vi "1.Primary Interface.vi"() -> ()   [LabVIEW 2020]
uses:
  UnderAutomation.UniversalRobots/UnderAutomation.UniversalRobots.lvlib
  C:/Users/fg/Documents/UniversalRobots.vi/LabVIEW_2024/UnderAutomation.UniversalRobots/lib/UnderAutomation.UniversalRobots.dll
  LabVIEW_2024/UnderAutomation.UniversalRobots/lib/UnderAutomation.UniversalRobots.dll
panel:
  out "UR Robot":refnum<k24>
  out "PrimaryInterface":refnum<k24>
  out "Connected":bool
  in  "Tab Control":T1(tab)
  in  "Disconnect":bool
  in  "Test":bool
  in  "Key":string
  in  "Licensee":string
  in  "Connect":bool
  in  "IP":string caption="Robot IP Address"
  out "License state":string
  out "Connect error":string
  in  "Script":string
  in  "Send":bool
  out "Variables":T2(array[cluster])
  out "CartesianInfo":T3
  out "ForceModeData":T4
  out "JointData":T5
  out "ToolData":T6
  out "AdditionalInfo":T7
  out "ToolCommunicationInfo":T8
  out "MasterboardData":T9
  out "ToolModeInfo":T10
  out "RobotModeData":T11
  out "TextMessage":cluster{"TextMessage":string}
  out "KeyMessage":T12
  out "PopupMessage":T13
  out "RuntimeExceptionMessage":T14
  out "KinematicsInfo":T15
  out "CalibrationData":T16
  out "SingularityInfo":T17
  out "ConfigurationData":T18
  out "Version":T19
  in  "stop":bool
  # "UnderAutomation"
  # "https://underautomation.com/universal-robots"
  # "+"
  # "LabVIEW demo app for remote control and monitoring of your Universal Robots cobot"
  # "Connect to robot"
  # "2. Ensure you have a trial or lifetime valid license"
  # "1. Set UR cobot address"
  # "This is a commercial library, you have a 30-day trial period. But you can use it forever if you buy a perpetual licence for your company (regardless of the number of robot, applications or developers)."
  # "If you have a license :"
  # "2. Connect to the robot"
  # "Send script"
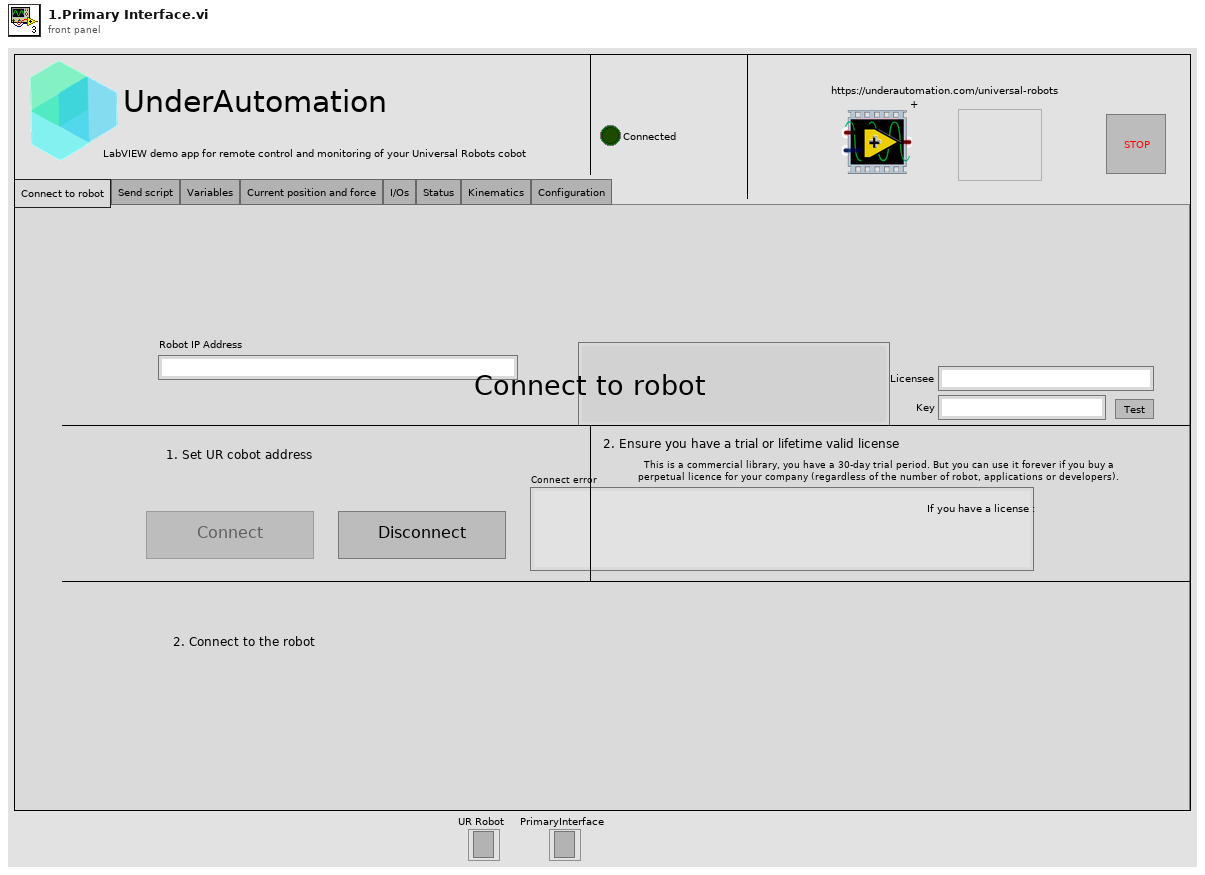
[diagram p1: front panel]
types:
  T1 = enum32{"Connect to robot", "Send script", "Variables", "Current position and force", "I/Os", "Status", "Kinematics", "Configuration"}
  T2 = cluster{"Name":string, "Milliseconds":i32, "Type":i32, "BoolValue":bool, "FloatValue":sgl, "IntValue":i32, "StringValue":string, "PoseValue":cluster{"X":dbl, "Y":dbl, "Z":dbl, "Rx":dbl, "Ry":dbl, "Rz":dbl}}[]
  T3 = cluster{"X":dbl, "Y":dbl, "Z":dbl, "Rx":dbl, "Ry":dbl, "Rz":dbl, "TCPOffsetX":dbl, "TCPOffsetY":dbl, "TCPOffsetZ":dbl, "TCPOffsetRX":dbl, "TCPOffsetRY":dbl, "TCPOffsetRZ":dbl}
  T4 = cluster{"X":dbl, "Y":dbl, "Z":dbl, "Rx":dbl, "Ry":dbl, "Rz":dbl, "RobotDexterity":dbl}
  T5 = cluster{"Base":cluster{"ActualSpeed":dbl, "Current":sgl, "JointMode":u8, "Position":dbl, "TargetPosition":dbl, "Temperature":sgl, "Voltage":sgl}, "Shoulder":cluster{"ActualSpeed":dbl, "Current":sgl, "JointMode":u8, "Position":dbl, "TargetPosition":dbl, "Temperature":sgl, "Voltage":sgl}, "Elbow":cluster{"ActualSpeed":dbl, "Current":sgl, "JointMode":u8, "Position":dbl, "TargetPosition":dbl, "Temperature":sgl, "Voltage":sgl}, "Wrist1":cluster{"ActualSpeed":dbl, "Current":sgl, "JointMode":u8, "Position":dbl, "TargetPosition":dbl, "Temperature":sgl, "Voltage":sgl}, "Wrist2":cluster{"ActualSpeed":dbl, "Current":sgl, "JointMode":u8, "Position":dbl, "TargetPosition":dbl, "Temperature":sgl, "Voltage":sgl}, "Wrist3":cluster{"ActualSpeed":dbl, "Current":sgl, "JointMode":u8, "Position":dbl, "TargetPosition":dbl, "Temperature":sgl, "Voltage":sgl}}
  T6 = cluster{"AnalogInput2":dbl, "AnalogInput3":dbl, "AnalogInputRange2":i32, "AnalogInputRange3":i32, "ToolCurrent":sgl, "ToolMode":u8, "ToolOutputVoltage":i8, "ToolTemperature":sgl, "ToolVoltage48V":sgl}
  T7 = cluster{"FreedriveButtonEnabled":bool, "FreedriveButtonPressed":bool, "IOEnabledFreedrive":bool}
  T8 = cluster{"BaudRate":i32, "Parity":i32, "RxIdleChars":sgl, "TxIdleChars":sgl, "ToolCommunicationIsEnabled":bool, "StopBits":i32}
  T9 = cluster{"AnalogInput0":dbl, "AnalogInput1":dbl, "AnalogInputRange0":i32, "AnalogInputRange1":i32, "AnalogOutput0":dbl, "AnalogOutput1":dbl, "AnalogOutputDomain0":i32, "AnalogOutputDomain1":i32, "DigitalInputs":cluster{"Configurable0":bool, "Configurable1":bool, "Configurable2":bool, "Configurable3":bool, "Configurable4":bool, "Configurable5":bool, "Configurable6":bool, "Configurable7":bool, "Digital0":bool, "Digital1":bool, "Digital2":bool, "Digital3":bool, "Digital4":bool, "Digital5":bool, "Digital6":bool, "Digital7":bool, "ToolDigital0":bool, "ToolDigital1":bool, "Value":i32}, "DigitalOutputs":cluster{"Configurable0":bool, "Configurable1":bool, "Configurable2":bool, "Configurable3":bool, "Configurable4":bool, "Configurable5":bool, "Configurable6":bool, "Configurable7":bool, "Digital0":bool, "Digital1":bool, "Digital2":bool, "Digital3":bool, "Digital4":bool, "Digital5":bool, "Digital6":bool, "Digital7":bool, "ToolDigital0":bool, "ToolDigital1":bool, "Value":i32}, "Euromap67Installed":i8, "EuromapCurrent":sgl, "EuromapInputBits":i32, "EuromapOutputBits":i32, "EuromapVoltage":sgl, "InReducedMode":u8, "MasterboardTemperature":sgl, "MasterIOCurrent":sgl, "OperationalModeSelectorInput":u8, "RobotCurrent":sgl, "RobotVoltage48V":sgl, "Safetymode":u8, "ThreePositionEnablingDeviceInput":u8}
  T10 = cluster{"DigitalOutputMode0":i32, "DigitalOutputMode1":i32, "OutputMode":i32}
  T11 = cluster{"ControlMode":i32, "EmergencyStopped":bool, "PhysicalRobotConnected":bool, "ProgramPaused":bool, "ProgramRunning":bool, "ProtectiveStopped":bool, "RealRobotEnabled":bool, "RobotMode":i32, "RobotPowerOn":bool, "SpeedScaling":dbl, "TargetSpeedFraction":dbl, "TargetSpeedFractionLimit":dbl, "TotalMilliseconds":dbl}
  T12 = cluster{"KeyTextMessage":string, "RobotMessageArgument":i32, "RobotMessageCode":i32, "RobotMessageTitle":string}
  T13 = cluster{"Blocking":bool, "Error":bool, "PopupMessageTitle":string, "PopupTextMessage":string, "RequestedType":i32, "RequestId":u32, "Warning":bool}
  T14 = cluster{"RuntimeExceptionTextMessage":string, "ScriptColumnNumber":i32, "ScriptLineNumber":i32}
  T15 = cluster{"Base":cluster{"Checksum":i32, "DHa":dbl, "Dhalpha":dbl, "DHd":dbl, "DHtheta":dbl}, "Shoulder":cluster{"Checksum":i32, "DHa":dbl, "Dhalpha":dbl, "DHd":dbl, "DHtheta":dbl}, "Elbow":cluster{"Checksum":i32, "DHa":dbl, "Dhalpha":dbl, "DHd":dbl, "DHtheta":dbl}, "Wrist1":cluster{"Checksum":i32, "DHa":dbl, "Dhalpha":dbl, "DHd":dbl, "DHtheta":dbl}, "Wrist2":cluster{"Checksum":i32, "DHa":dbl, "Dhalpha":dbl, "DHd":dbl, "DHtheta":dbl}, "Wrist3":cluster{"Checksum":i32, "DHa":dbl, "Dhalpha":dbl, "DHd":dbl, "DHtheta":dbl}, "CalibrationStatus":i32}
  T16 = cluster{"Fx":dbl, "Fy":dbl, "Fz":dbl, "Frx":dbl, "Fry":dbl, "Frz":dbl}
  T17 = cluster{"SingularitySeverity":u8, "SingularityType":u8}
  T18 = cluster{"AJointDefault":dbl, "AToolDefault":dbl, "ControllerBoxType":i32, "EqRadius":dbl, "MasterboardVersion":i32, "RobotSubType":i32, "RobotType":i32, "VJointDefault":dbl, "VToolDefault":dbl, "Base":cluster{"DHa":dbl, "DHalpha":dbl, "DHd":dbl, "DHtheta":dbl, "JointMaxAcceleration":dbl, "JointMaxLimit":dbl, "JointMaxSpeed":dbl, "JointMinLimit":dbl}, "Shoulder":cluster{"DHa":dbl, "DHalpha":dbl, "DHd":dbl, "DHtheta":dbl, "JointMaxAcceleration":dbl, "JointMaxLimit":dbl, "JointMaxSpeed":dbl, "JointMinLimit":dbl}, "Elbow":cluster{"DHa":dbl, "DHalpha":dbl, "DHd":dbl, "DHtheta":dbl, "JointMaxAcceleration":dbl, "JointMaxLimit":dbl, "JointMaxSpeed":dbl, "JointMinLimit":dbl}, "Wrist1":cluster{"DHa":dbl, "DHalpha":dbl, "DHd":dbl, "DHtheta":dbl, "JointMaxAcceleration":dbl, "JointMaxLimit":dbl, "JointMaxSpeed":dbl, "JointMinLimit":dbl}, "Wrist2":cluster{"DHa":dbl, "DHalpha":dbl, "DHd":dbl, "DHtheta":dbl, "JointMaxAcceleration":dbl, "JointMaxLimit":dbl, "JointMaxSpeed":dbl, "JointMinLimit":dbl}, "Wrist3":cluster{"DHa":dbl, "DHalpha":dbl, "DHd":dbl, "DHtheta":dbl, "JointMaxAcceleration":dbl, "JointMaxLimit":dbl, "JointMaxSpeed":dbl, "JointMinLimit":dbl}}
  T19 = cluster{"MajorVersion":u8, "MinorVersion":u8, "BugfixVersion":i32, "BuildNumber":i32, "BuildDate":string, "ProjectName":string}
  T20 = enum8{"Enabled", "Disabled", "Disabled and Grayed Out"}
  T21 = cluster{"AdditionalInfo":cluster{"FreedriveButtonEnabled":bool, "FreedriveButtonPressed":bool, "IOEnabledFreedrive":bool}, "CalibrationData":cluster{"Fx":dbl, "Fy":dbl, "Fz":dbl, "Frx":dbl, "Fry":dbl, "Frz":dbl}, "CartesianInfo":cluster{"X":dbl, "Y":dbl, "Z":dbl, "Rx":dbl, "Ry":dbl, "Rz":dbl, "TCPOffsetX":dbl, "TCPOffsetY":dbl, "TCPOffsetZ":dbl, "TCPOffsetRX":dbl, "TCPOffsetRY":dbl, "TCPOffsetRZ":dbl}, "ConfigurationData":cluster{"AJointDefault":dbl, "AToolDefault":dbl, "ControllerBoxType":i32, "EqRadius":dbl, "MasterboardVersion":i32, "RobotSubType":i32, "RobotType":i32, "VJointDefault":dbl, "VToolDefault":dbl, "Base":cluster{"DHa":dbl, "DHalpha":dbl, "DHd":dbl, "DHtheta":dbl, "JointMaxAcceleration":dbl, "JointMaxLimit":dbl, "JointMaxSpeed":dbl, "JointMinLimit":dbl}, "Shoulder":cluster{"DHa":dbl, "DHalpha":dbl, "DHd":dbl, "DHtheta":dbl, "JointMaxAcceleration":dbl, "JointMaxLimit":dbl, "JointMaxSpeed":dbl, "JointMinLimit":dbl}, "Elbow":cluster{"DHa":dbl, "DHalpha":dbl, "DHd":dbl, "DHtheta":dbl, "JointMaxAcceleration":dbl, "JointMaxLimit":dbl, "JointMaxSpeed":dbl, "JointMinLimit":dbl}, "Wrist1":cluster{"DHa":dbl, "DHalpha":dbl, "DHd":dbl, "DHtheta":dbl, "JointMaxAcceleration":dbl, "JointMaxLimit":dbl, "JointMaxSpeed":dbl, "JointMinLimit":dbl}, "Wrist2":cluster{"DHa":dbl, "DHalpha":dbl, "DHd":dbl, "DHtheta":dbl, "JointMaxAcceleration":dbl, "JointMaxLimit":dbl, "JointMaxSpeed":dbl, "JointMinLimit":dbl}, "Wrist3":cluster{"DHa":dbl, "DHalpha":dbl, "DHd":dbl, "DHtheta":dbl, "JointMaxAcceleration":dbl, "JointMaxLimit":dbl, "JointMaxSpeed":dbl, "JointMinLimit":dbl}}, "ForceModeData":cluster{"X":dbl, "Y":dbl, "Z":dbl, "Rx":dbl, "Ry":dbl, "Rz":dbl, "RobotDexterity":dbl}, "JointData":cluster{"Base":cluster{"ActualSpeed":dbl, "Current":sgl, "JointMode":u8, "Position":dbl, "TargetPosition":dbl, "Temperature":sgl, "Voltage":sgl}, "Shoulder":cluster{"ActualSpeed":dbl, "Current":sgl, "JointMode":u8, "Position":dbl, "TargetPosition":dbl, "Temperature":sgl, "Voltage":sgl}, "Elbow":cluster{"ActualSpeed":dbl, "Current":sgl, "JointMode":u8, "Position":dbl, "TargetPosition":dbl, "Temperature":sgl, "Voltage":sgl}, "Wrist1":cluster{"ActualSpeed":dbl, "Current":sgl, "JointMode":u8, "Position":dbl, "TargetPosition":dbl, "Temperature":sgl, "Voltage":sgl}, "Wrist2":cluster{"ActualSpeed":dbl, "Current":sgl, "JointMode":u8, "Position":dbl, "TargetPosition":dbl, "Temperature":sgl, "Voltage":sgl}, "Wrist3":cluster{"ActualSpeed":dbl, "Current":sgl, "JointMode":u8, "Position":dbl, "TargetPosition":dbl, "Temperature":sgl, "Voltage":sgl}}, "KeyMessage":cluster{"KeyTextMessage":string, "RobotMessageArgument":i32, "RobotMessageCode":i32, "RobotMessageTitle":string}, "KinematicsInfo":cluster{"Base":cluster{"Checksum":i32, "DHa":dbl, "Dhalpha":dbl, "DHd":dbl, "DHtheta":dbl}, "Shoulder":cluster{"Checksum":i32, "DHa":dbl, "Dhalpha":dbl, "DHd":dbl, "DHtheta":dbl}, "Elbow":cluster{"Checksum":i32, "DHa":dbl, "Dhalpha":dbl, "DHd":dbl, "DHtheta":dbl}, "Wrist1":cluster{"Checksum":i32, "DHa":dbl, "Dhalpha":dbl, "DHd":dbl, "DHtheta":dbl}, "Wrist2":cluster{"Checksum":i32, "DHa":dbl, "Dhalpha":dbl, "DHd":dbl, "DHtheta":dbl}, "Wrist3":cluster{"Checksum":i32, "DHa":dbl, "Dhalpha":dbl, "DHd":dbl, "DHtheta":dbl}, "CalibrationStatus":i32}, "MasterboardData":cluster{"AnalogInput0":dbl, "AnalogInput1":dbl, "AnalogInputRange0":i32, "AnalogInputRange1":i32, "AnalogOutput0":dbl, "AnalogOutput1":dbl, "AnalogOutputDomain0":i32, "AnalogOutputDomain1":i32, "DigitalInputs":cluster{"Configurable0":bool, "Configurable1":bool, "Configurable2":bool, "Configurable3":bool, "Configurable4":bool, "Configurable5":bool, "Configurable6":bool, "Configurable7":bool, "Digital0":bool, "Digital1":bool, "Digital2":bool, "Digital3":bool, "Digital4":bool, "Digital5":bool, "Digital6":bool, "Digital7":bool, "ToolDigital0":bool, "ToolDigital1":bool, "Value":i32}, "DigitalOutputs":cluster{"Configurable0":bool, "Configurable1":bool, "Configurable2":bool, "Configurable3":bool, "Configurable4":bool, "Configurable5":bool, "Configurable6":bool, "Configurable7":bool, "Digital0":bool, "Digital1":bool, "Digital2":bool, "Digital3":bool, "Digital4":bool, "Digital5":bool, "Digital6":bool, "Digital7":bool, "ToolDigital0":bool, "ToolDigital1":bool, "Value":i32}, "Euromap67Installed":i8, "EuromapCurrent":sgl, "EuromapInputBits":i32, "EuromapOutputBits":i32, "EuromapVoltage":sgl, "InReducedMode":u8, "MasterboardTemperature":sgl, "MasterIOCurrent":sgl, "OperationalModeSelectorInput":u8, "RobotCurrent":sgl, "RobotVoltage48V":sgl, "Safetymode":u8, "ThreePositionEnablingDeviceInput":u8}, "PopupMessage":cluster{"Blocking":bool, "Error":bool, "PopupMessageTitle":string, "PopupTextMessage":string, "RequestedType":i32, "RequestId":u32, "Warning":bool}, "RobotModeData":cluster{"ControlMode":i32, "EmergencyStopped":bool, "PhysicalRobotConnected":bool, "ProgramPaused":bool, "ProgramRunning":bool, "ProtectiveStopped":bool, "RealRobotEnabled":bool, "RobotMode":i32, "RobotPowerOn":bool, "SpeedScaling":dbl, "TargetSpeedFraction":dbl, "TargetSpeedFractionLimit":dbl, "TotalMilliseconds":dbl}, "RuntimeExceptionMessage":cluster{"RuntimeExceptionTextMessage":string, "ScriptColumnNumber":i32, "ScriptLineNumber":i32}, "SingularityInfo":cluster{"SingularitySeverity":u8, "SingularityType":u8}, "TextMessage":cluster{"TextMessage":string}, "ToolCommunicationInfo":cluster{"BaudRate":i32, "Parity":i32, "RxIdleChars":sgl, "TxIdleChars":sgl, "ToolCommunicationIsEnabled":bool, "StopBits":i32}, "ToolData":cluster{"AnalogInput2":dbl, "AnalogInput3":dbl, "AnalogInputRange2":i32, "AnalogInputRange3":i32, "ToolCurrent":sgl, "ToolMode":u8, "ToolOutputVoltage":i8, "ToolTemperature":sgl, "ToolVoltage48V":sgl}, "ToolModeInfo":cluster{"DigitalOutputMode0":i32, "DigitalOutputMode1":i32, "OutputMode":i32}, "Version":cluster{"MajorVersion":u8, "MinorVersion":u8, "BugfixVersion":i32, "BuildNumber":i32, "BuildDate":string, "ProjectName":string}}
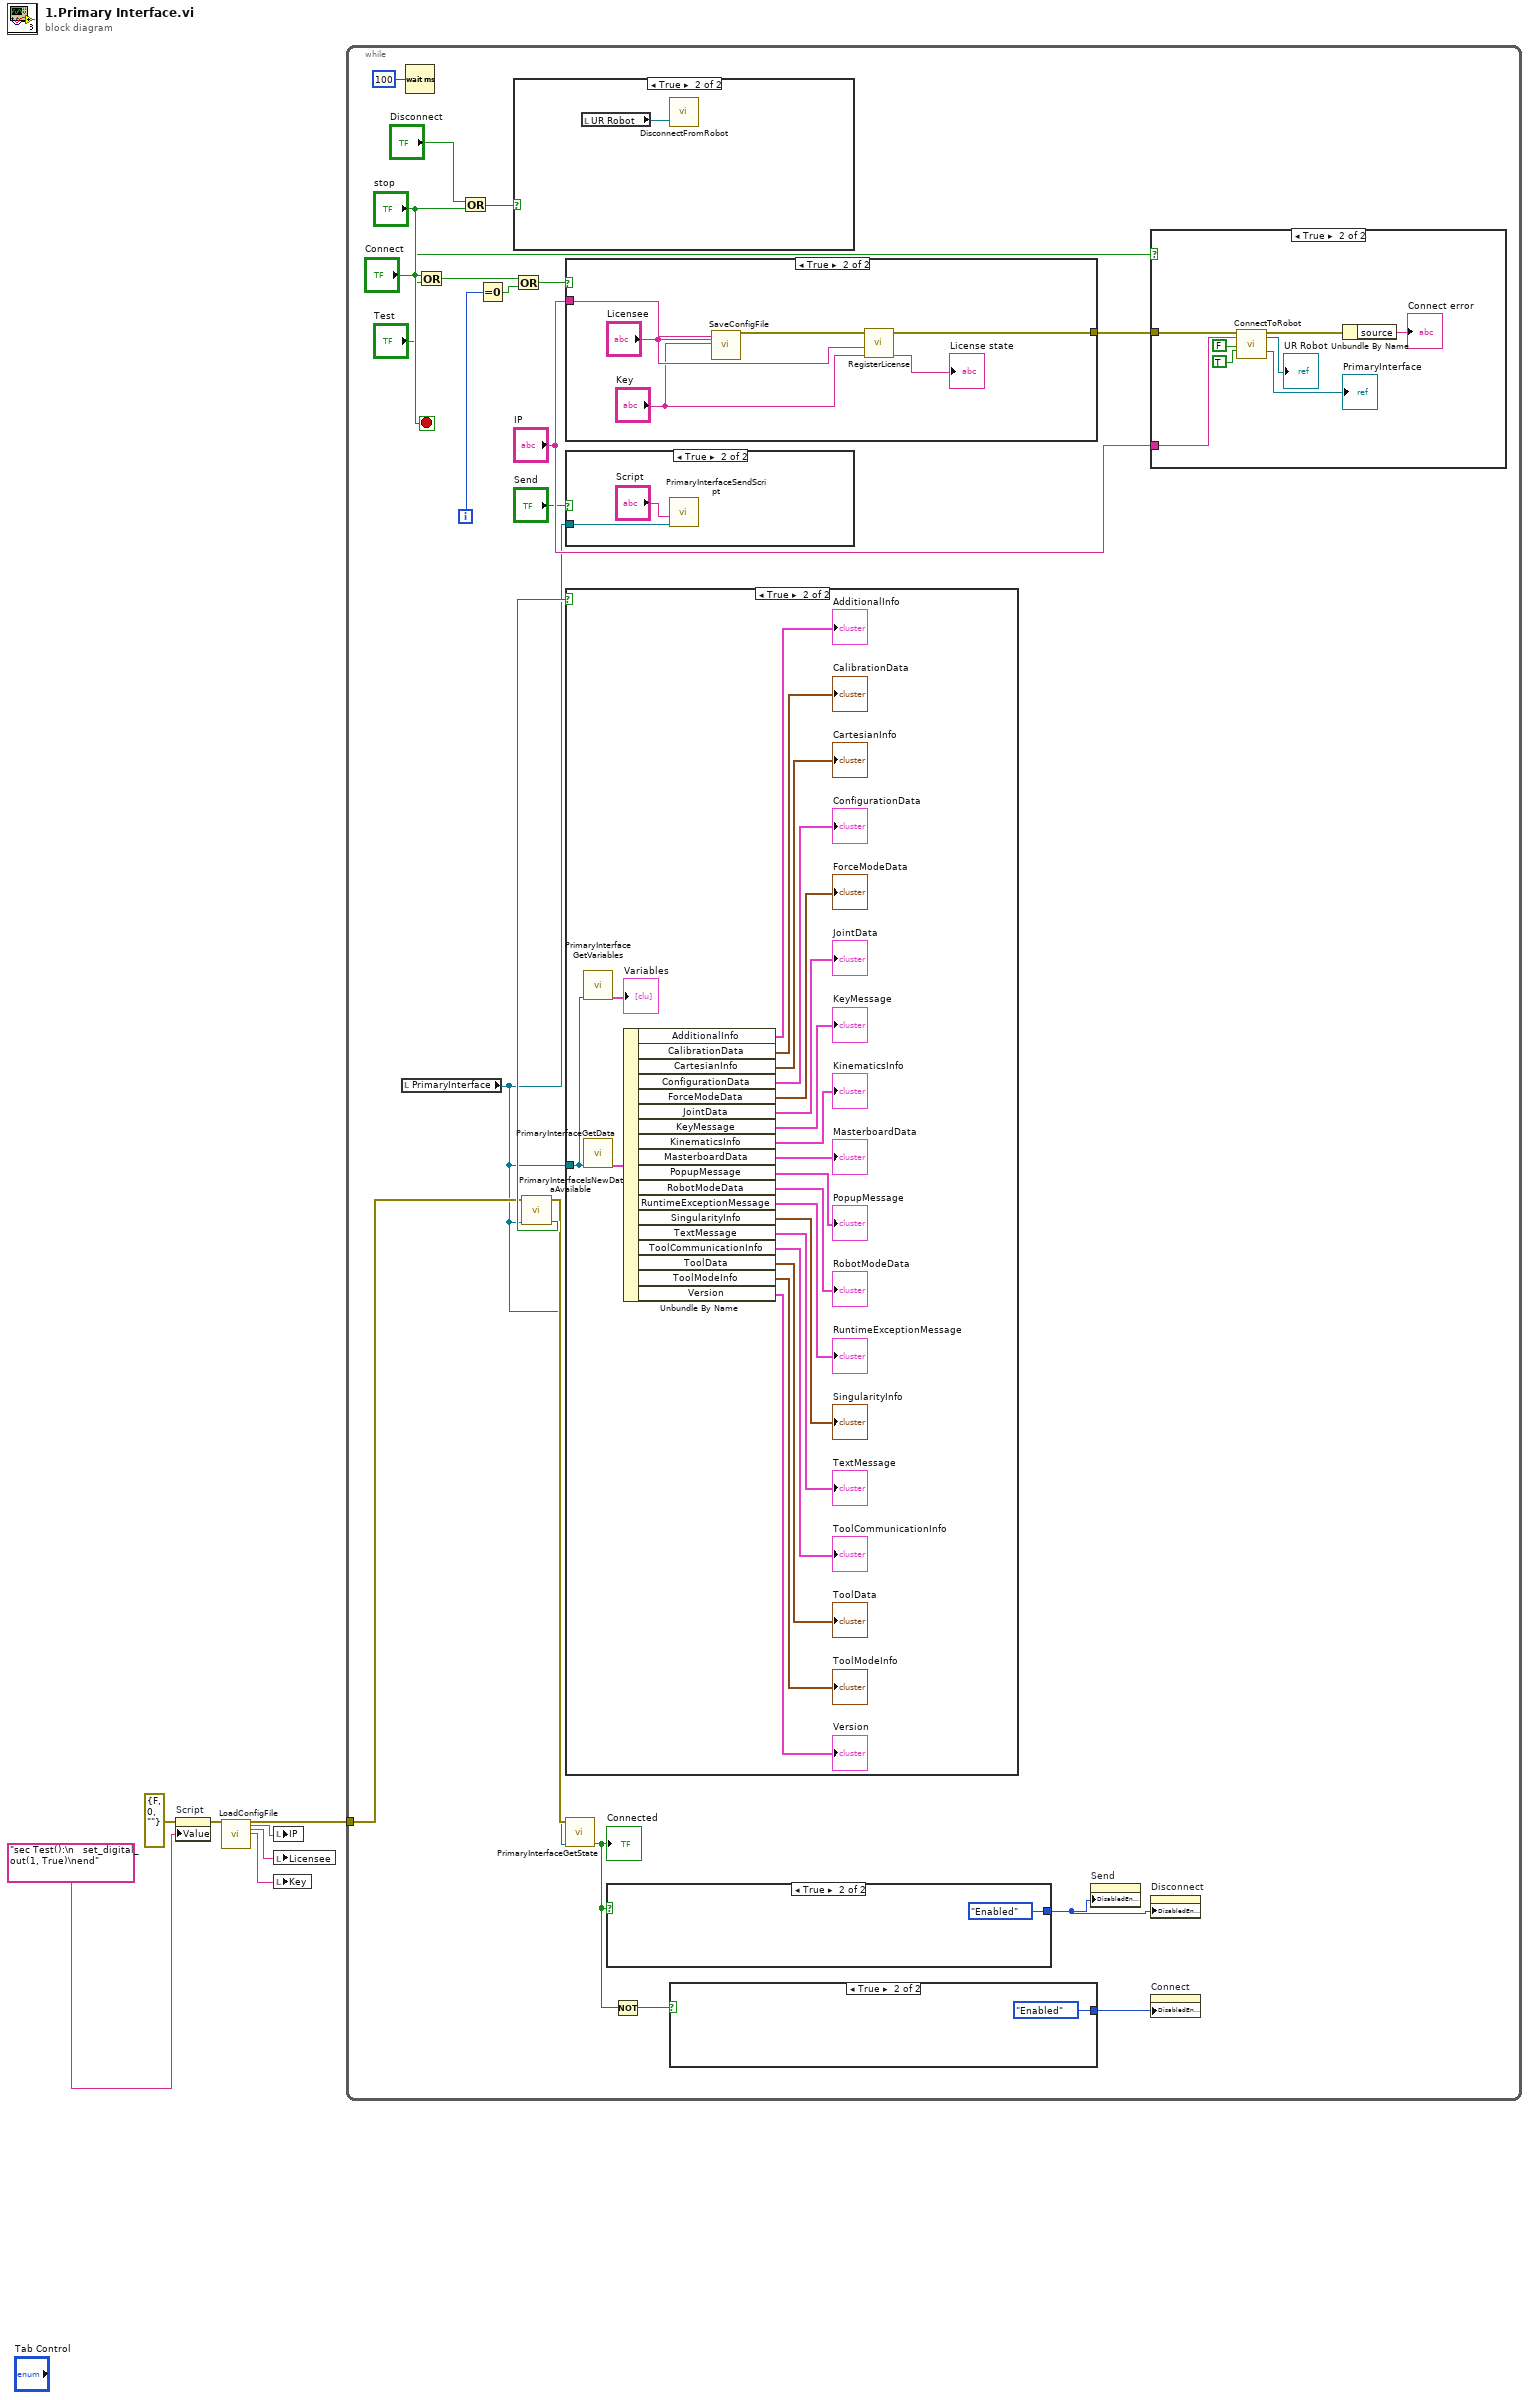
[diagram p0: block diagram]
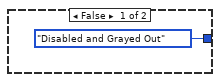
[diagram p3: hidden frame]
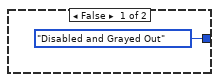
[diagram p4: hidden frame]
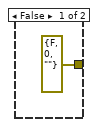
[diagram p5: hidden frame]
diagram:
  n1 = property on="Script" class="Str"(error in=errorcluster {"status"=FALSE, "code"=0, "source"=""} ("error in (no error)"), "Value"="sec Test():\n   set_digital_out(1, True)\nend" ("Script")) -> (error out=w2:errorcluster)  [unwired: 1 in, 1 out]
  n2 = call "LoadConfigFile.vi"("error in (no error)"=w2) -> ("error out"=w4:errorcluster, "IP"=w5:string, "Licensee"=w7:string, "Key"=w6:string)  [unwired: 21 in, 2 out]
  n3 = local write "IP"(w5) -> ()
  n4 = local write "Licensee"(w7) -> ()
  n5 = local write "Key"(w6) -> ()
  n6 = while {
    tunnel: w4 -> [w16]
    i -> [w21]
    stop <- "stop" stop-if-true
    n7 = local read "PrimaryInterface"() -> (w9:refnum<k24>)
    n8 = Wait (ms)(milliseconds to wait=u32 100) -> ()  [unwired: 1 out]
    n9 = Or(x="Connect", y="Test") -> (x .or. y?=w19:bool)
    n10 = Or(x="Disconnect", y="stop") -> (x .or. y?=w26:bool)
    n11 = Equal To 0?(x=w21) -> (x = 0?=w20:bool)
    n12 = case shown="True" w26 {
      frame False {
      }
      frame True {
        n13 = local read "UR Robot"() -> (w71:refnum<k24>)
        n14 = call "DisconnectFromRobot.vi"("UR Robot"=w71) -> ()  [unwired: 2 in, 1 out]
      }
    }
    n15 = Or(x=w19, y=w20) -> (x .or. y?=w18:bool)
    n16 = call "PrimaryInterfaceIsNewDataAvailable.vi"("PrimaryInterface"=w9, "error in"=w16) -> ("Data available"=w25:bool, "error out"=w11:errorcluster)  [unwired: 8 in]
    n17 = case shown="True" w18 {
      tunnel: [errorcluster {"status"=FALSE, "code"=0, "source"=""} ("error out") w40] -> w17
      tunnel: "IP" -> [_ w37]
      frame False {
      }
      frame True {
        n18 = call "SaveConfigFile.vi"("IP"=w37, "Licensee"="Licensee", "Key"="Key") -> ("error out"=w36:errorcluster)  [unwired: 24 in]
        n19 = call "RegisterLicense.vi"("key"="Key", "licensee"="Licensee", "error in"=w36) -> ("State message"=→"License state":string, "error out"=w40:errorcluster)  [unwired: 5 in, 1 out]
      }
    }
    n20 = case shown="True" "Send" {
      tunnel: w9 -> [_ w29]
      frame False {
      }
      frame True {
        n21 = call "PrimaryInterfaceSendScript.vi"("PrimaryInterface"=w29, "script"="Script") -> ()  [unwired: 9 in, 1 out]
      }
    }
    n22 = case shown="True" w25 {
      tunnel: w9 -> [_ w51]
      frame False {
      }
      frame True {
        n23 = call "PrimaryInterfaceGetVariables.vi"("PrimaryInterface"=w51) -> ("Variables"=→"Variables":T2)  [unwired: 9 in, 1 out]
        n24 = call "PrimaryInterfaceGetData.vi"("PrimaryInterface"=w51) -> ("Data"=w52:T21)  [unwired: 9 in, 1 out]
        n25 = Unbundle By Name(w52) -> ("AdditionalInfo"=→"AdditionalInfo":T7, "CalibrationData"=→"CalibrationData":T16, "CartesianInfo"=→"CartesianInfo":T3, "ConfigurationData"=→"ConfigurationData":T18, "ForceModeData"=→"ForceModeData":T4, "JointData"=→"JointData":T5, "KeyMessage"=→"KeyMessage":T12, "KinematicsInfo"=→"KinematicsInfo":T15, "MasterboardData"=→"MasterboardData":T9, "PopupMessage"=→"PopupMessage":T13, "RobotModeData"=→"RobotModeData":T11, "RuntimeExceptionMessage"=→"RuntimeExceptionMessage":T14, "SingularityInfo"=→"SingularityInfo":T17, "TextMessage"=→"TextMessage":cluster{"TextMessage":string}, "ToolCommunicationInfo"=→"ToolCommunicationInfo":T8, "ToolData"=→"ToolData":T6, "ToolModeInfo"=→"ToolModeInfo":T10, "Version"=→"Version":T19)
      }
    }
    n26 = call "PrimaryInterfaceGetState.vi"("PrimaryInterface"=w9, "error in"=w11) -> ("Connected"=w13:bool)  [unwired: 8 in, 1 out]
    "Connected" <- w13
    n27 = case shown="True" w13 {
      tunnel: [T20."Disabled and Grayed Out" ("Disabled") T20."Enabled" ("Disabled")] -> w8
      frame False {
      }
      frame True {
      }
    }
    n28 = Not(x=w13) -> (.not. x?=w14:bool)
    n29 = case shown="True" w14 {
      tunnel: [T20."Disabled and Grayed Out" ("Disabled") T20."Enabled" ("Disabled")] -> w12
      frame False {
      }
      frame True {
      }
    }
    n30 = property on="Send" class="Bool"("DisabledEnum"=w8) -> ()  [unwired: 2 in, 2 out]
    n31 = case shown="True" "Connect" {
      tunnel: w17 -> [_ w43]
      tunnel: "IP" -> [_ w42]
      frame False {
      }
      frame True {
        n32 = call "ConnectToRobot.vi"("error in"=w43, "ip"=w42, "Enable Dashboard"=FALSE ("Enable Primary Interface"), "Enable Primary Interface"=TRUE) -> ("error out"=w47:errorcluster, "UR Robot"=→"UR Robot":refnum<k24>, "PrimaryInterface"=→"PrimaryInterface":refnum<k24>)  [unwired: 10 in, 3 out]
        n33 = Unbundle By Name(w47) -> ("source"=→"Connect error":string)
      }
    }
    n34 = property on="Disconnect" class="Bool"("DisabledEnum"=w8) -> ()  [unwired: 2 in, 2 out]
    n35 = property on="Connect" class="Bool"("DisabledEnum"=w12) -> ()  [unwired: 2 in, 2 out]
  }
